vi "FAMM-service.vi"(8 "error in (no error)":errorcluster, 11 "FAMM_in":refnum<class "FAMM.lvclass">) -> (0 "error out":errorcluster, 3 "FAMM_out":refnum<class "FAMM.lvclass">)   [LabVIEW 2020, in "Sgraph_lib_V1.lvlib" / "FAMM.lvclass"]
doc: "The FAMM server is instantiated by Gserver\nThe FAMM server will process all queue driven commands to read and write from memory, and via the FAMM server access memory or database content.\n\nWhether RAM or Database content is accessed is decided by the FAMM service. Database content is not intended to be accessed directly without using the FAMM service."
uses:
  FAMM.lvclass
  Gserver/controls/Typedef_Gviewer-Query.ctl
  Gserver/controls/Typedef_QueryType.ctl
  HISW/controls/typedef-DAQ-datagram.ctl
  HISW/controls/typedef-Qtype.ctl
  FAMM.lvclass/FAMM.ctl
  controls/FAMMrequest.ctl
  Gview/controls/Typedef_Live.ctl
  DBAL/controls/DBAL_TAGpropEdit.ctl
  Common/controls/typedef_com_TagProp.ctl
  Builds/Sgraph_lib_V1.lvlib
  Gview/Gviewer.lvclass
  DBAL/DBAL.lvclass
  Gserver/Gserver.lvclass
panel:
  in  "OS_type":string="undefined"
  in  "Database_path":path=path "D:/Sgraph_database"
  out "Layers":i32
  out "sec resolution":dbl format="%#_3p"
  out "37x37":picture
  in  "DAQ-Queue":refnum<queue>
  in  "Gserver-Queue":refnum<queue>
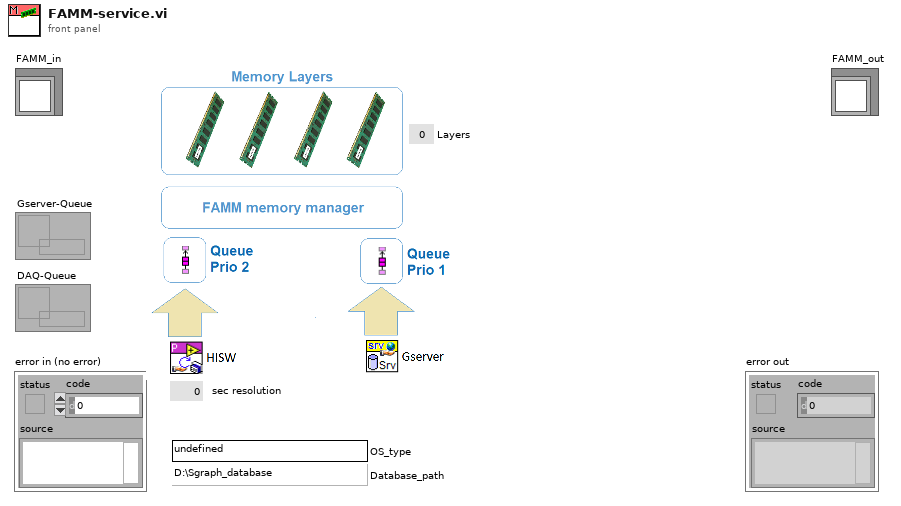
[diagram p1: front panel]
types:
  T1 = typedef "Sgraph_lib_V1.lvlib/FAMM.lvclass/FAMMrequest.ctl" = cluster{"Tags":string[], "Time-Start":timestamp, "Time-End":timestamp, "Live":T2, "TimeSpan":dbl, "DisplayResolution":i32}
  T2 = typedef "Sgraph_lib_V1.lvlib/Gviewer.lvclass/Typedef_Live.ctl" = enum16{"Live View", "Freeze"}
  T3 = typedef "Sgraph_lib_V1.lvlib/DBAL.lvclass/DBAL_TAGpropEdit.ctl" = cluster{"TAG":string, "Qtype":string, "TAGprop":T4}
  T4 = typedef "Sgraph_lib_V1.lvlib/typedef_com_TagProp.ctl" = cluster{"Description":string, "EngUnits":string, "RangeH":dbl, "RangeL":dbl, "Resolution":i32, "Obsolete":bool, "ChangeDate":timestamp, "ChangeSource":string, "ChangeReason":string, "TagFunc":u32}
  T5 = typedef "typedef_FAMM_Query.ctl" = cluster{"Time Stamp":timestamp, "FAMM-function":T6, "Source":string, "Data":variant}
  T6 = typedef "Sgraph_lib_V1.lvlib/typedef-functions.ctl" = enum16{"PAQ-request", "PAQ-taglist-request", "WAQ-request", "EAQ-request", "TAG-based-request", "PAQ-MemoryMap", "Update-TAG-property", "Exit-FAMM"}
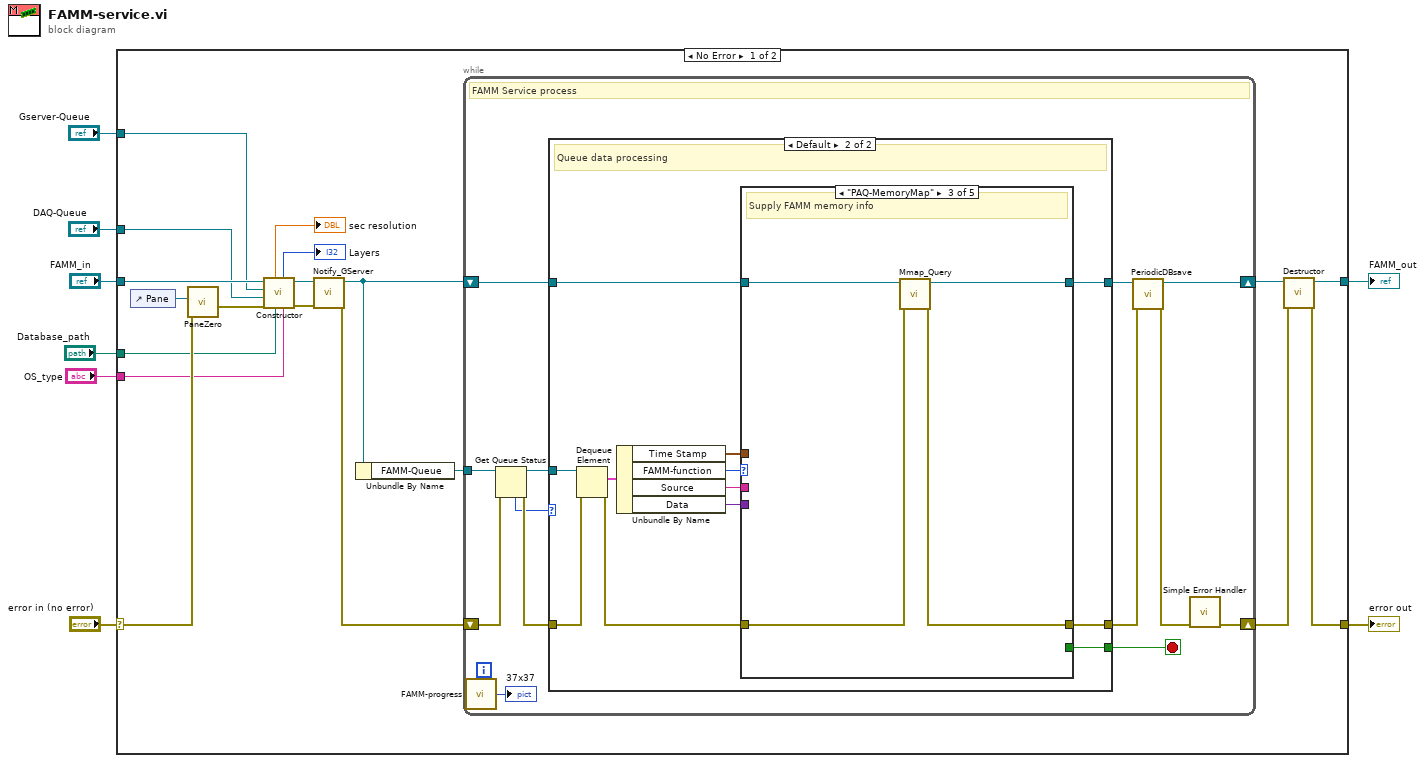
[diagram p0: block diagram]
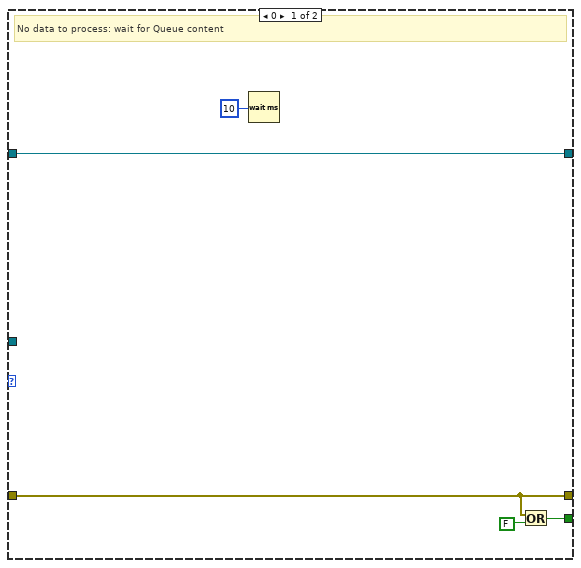
[diagram p2: hidden frame]
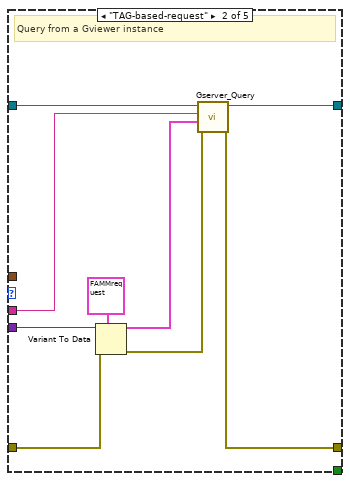
[diagram p4: hidden frame]
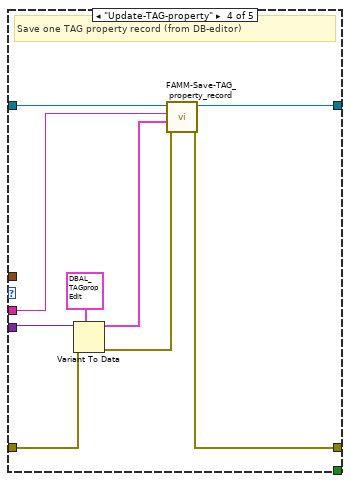
[diagram p5: hidden frame]
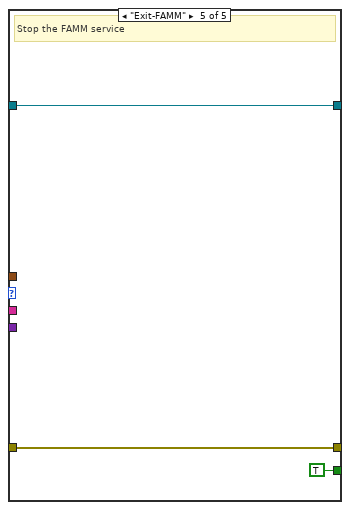
[diagram p6: hidden frame]
diagram:
  n1 = case shown="No Error" "error in (no error)" {
    selector: "error in (no error)" -> [w18 w86]
    tunnel: [w24 w86] -> w7
    tunnel: [w26 w85] -> w6
    tunnel: "FAMM_in" -> [w20 w85]
    tunnel: "Gserver-Queue" -> [w16 _]
    tunnel: "DAQ-Queue" -> [w14 _]
    tunnel: "Database_path" -> [w10 _]
    tunnel: "OS_type" -> [w9 _]
    frame No Error {
      n2 = control-ref of="Pane"() -> (w17:refnum<vi>)
      n3 = call "PaneZero.vi"("error in (no error)"=w18, "Pane"=w17) -> ("error out"=w19:errorcluster)  [unwired: 9 in]
      n4 = call "Constructor.vi"("OS_type"=w9, "Database_path"=w10, "error in (no error)"=w19, "DAQ-Queue"=w14, "Gserver-Queue"=w16, "FAMM in"=w20) -> ("error out"=w22:errorcluster, "FAMM out"=w23:refnum<class "FAMM.lvclass">, "Layers"=→"Layers":i32, "Resolution"=→"sec resolution":dbl)  [unwired: 2 in]
      n5 = call "Notify_GServer.vi"("error in (no error)"=w22, "FAMM in"=w23) -> ("error out"=w21:errorcluster, "FAMM out"=w13:refnum<class "FAMM.lvclass">)  [unwired: 8 in]
      n6 = Unbundle By Name(w13) -> ("FAMM-Queue"=w15:refnum<queue>)
      n7 = while {
        shift-right: [w32] -> w27
        shift-left: w13 -> [w33]
        shift-right: [w28] -> w25
        shift-left: w21 -> [w40]
        tunnel: w15 -> [w38]
        stop <- w35 stop-if-true
        # "FAMM Service process"
        n8 = call "FAMM-progress.vi"() -> ("37x37"=→"37x37":picture)  [unwired: 7 in]
        n9 = Get Queue Status(queue=w38, error in (no error)=w40) -> (queue out=w37:refnum<queue>, error out=w39:errorcluster, # elements in queue=w36:i32)  [unwired: 1 in, 5 out]
        n10 = case shown="Default" w36 {
          tunnel: [w41 w57] -> w30
          tunnel: w39 -> [w41 w50]
          tunnel: w33 -> [w43 w46]
          tunnel: [w43 w56] -> w31
          tunnel: w37 -> [_ w55]
          tunnel: [w44 w52] -> w35
          frame 0 {
            # "No data to process: wait for Queue content"
            n11 = Wait (ms)(milliseconds to wait=u32 10) -> ()  [unwired: 1 out]
            n12 = Or(x=w41, y=FALSE) -> (x .or. y?=w44:bool)
          }
          frame Default {
            # "Queue data processing"
            n13 = Dequeue Element(queue=w55, error in (no error)=w50) -> (element=w54:T5, error out=w51:errorcluster)  [unwired: 1 in, 2 out]
            n14 = Unbundle By Name(w54) -> ("Time Stamp"=w47:timestamp, "FAMM-function"=w53:T6, "Source"=w49:string, "Data"=w48:variant)
            n15 = case shown="\"PAQ-MemoryMap\"" w53 {
              tunnel: w46 -> [w59 w67 w71 w80 w82]
              tunnel: [w59 w68 w72 w81 w82] -> w56
              tunnel: w51 -> [w58 w63 w70 w76 w84]
              tunnel: [w58 w64 w69 w79 w84] -> w57
              tunnel: [_ _ _ _ TRUE] -> w52
              tunnel: w49 -> [_ w60 _ w73 _]
              tunnel: w48 -> [_ w66 _ w78 _]
              tunnel: w47 -> [_ _ _ _ _]
              frame Default {
                # "Not defined"
              }
              frame "TAG-based-request" {
                # "Query from a Gviewer instance"
                n16 = Variant To Data(error in=w63, type=T1 {"Tags"=["ch0001", "ch0002", "ch0003", "ch0004", "ch0005"], "Time-Start"=timestamp(3693712856.876272 s since 1904-01-01), "Time-End"=timestamp(3693716456.876272 s since 1904-01-01), "Live"=enum."Live View", "TimeSpan"=0.0, "DisplayResolution"=0} ("FAMM-request"), Variant=w66) -> (data=w61:T1, error out=w65:errorcluster)
                n17 = call "Gserver_Query.vi"("error in (no error)"=w65, "Query"=w61, "Requester"=w60, "FAMM in"=w67) -> ("error out"=w64:errorcluster, "FAMM out"=w68:refnum<class "FAMM.lvclass">)  [unwired: 6 in]
              }
              frame "PAQ-MemoryMap" {
                # "Supply FAMM memory info"
                n18 = call "Mmap_Query.vi"("error in (no error)"=w70, "FAMM in"=w71) -> ("error out"=w69:errorcluster, "FAMM out"=w72:refnum<class "FAMM.lvclass">)  [unwired: 8 in]
              }
              frame "Update-TAG-property" {
                # "Save one TAG property record (from DB-editor)"
                n19 = Variant To Data(error in=w76, type=T3 {"TAG"="", "Qtype"="", "TAGprop"={"Description"="", "EngUnits"="", "RangeH"=0.0, "RangeL"=0.0, "Resolution"=0, "Obsolete"=FALSE, "ChangeDate"=timestamp(0 s since 1904-01-01), "ChangeSource"="", "ChangeReason"="", "TagFunc"=0}} ("output cluster"), Variant=w78) -> (data=w74:T3, error out=w77:errorcluster)
                n20 = call "FAMM-Save-TAG_property_record.vi"("error in (no error)"=w77, "TAG-property"=w74, "Source"=w73, "FAMM in"=w80) -> ("error out"=w79:errorcluster, "FAMM out"=w81:refnum<class "FAMM.lvclass">)  [unwired: 6 in]
              }
              frame "Exit-FAMM" {
                # "Stop the FAMM service"
              }
            }
          }
        }
        n21 = call "PeriodicDBsave.vi"("error in (no error)"=w30, "FAMM in"=w31) -> ("error out"=w29:errorcluster, "FAMM out"=w32:refnum<class "FAMM.lvclass">)  [unwired: 8 in]
        n22 = call <vilib>:"Simple Error Handler.vi"("error in (no error)"=w29) -> ("error out"=w28:errorcluster)  [unwired: 4 in, 4 out]
      }
      n23 = call "Destructor.vi"("error in (no error)"=w25, "FAMM in"=w27) -> ("error out"=w24:errorcluster, "FAMM out"=w26:refnum<class "FAMM.lvclass">)  [unwired: 8 in]
    }
    frame Error {
    }
  }
  "error out" <- w7
  "FAMM_out" <- w6
